vi "Create.vi"(8 "error in (no error)":errorcluster, 10 "Subsystem Name (optional)":string, 11 "SMO":refnum<class "SMO.lvclass">) -> (0 "error out":errorcluster, 2 "SMO name":string, 3 "SMO out":refnum<class "SMO.lvclass">)   [LabVIEW 2013, in "SMO.lvclass"]
doc: "Constructor\n\nNote 01: This method is overridable by descendant\nNote 02: When overridden, Call Parent Method is required\n\n---------------------------------------------------------------\nJKI State Machine Objects™\nhttp://jki.net/state-machine-objects/\nCopyright (C) 2005-2015, JKI <info@jki.net>\nALL RIGHTS RESERVED"
uses:
  SMO.lvclass
  SMO.lvclass/SMO.ctl
  Typedefs/Process Error Notification--Cluster.ctl
  Typedefs/SMOState --Enum.ctl
  Registry/Registry-SMO.lvclass
  Support/Attribute.Identity/Attribute.Identity.lvclass
panel:
  # "For instructions on how to use the JKI State Machine Objects, examples and video tutorials, visit:\nhttp://jki.net/state-machine-objects/\n\nJKI State Machine Objects™\nhttp://jki.net/state-machine-objects/\nCopyright (C) 2005-2015, JKI <info@jki.net>\nALL RIGHTS RESERVED"
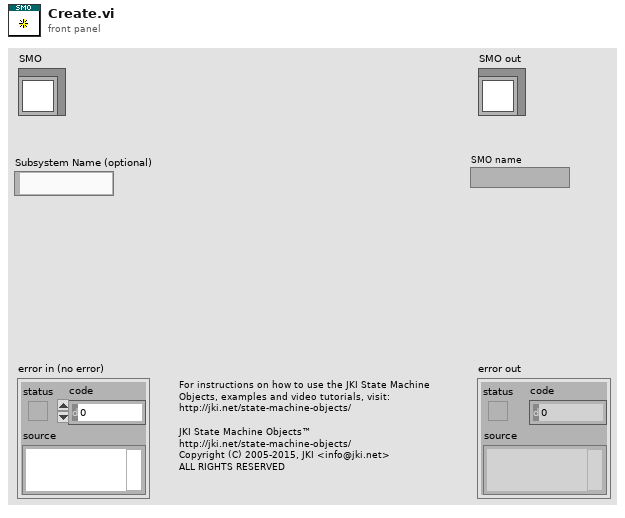
[diagram p1: front panel]
types:
  T1 = typedef "SMO.lvclass/SMOState --Enum.ctl" = enum16{"unknown", "Created", "Started", "Stopped"}
  T2 = typedef "SMO.lvclass/Process Error Notification--Cluster.ctl" = cluster{"error":errorcluster}
  T3 = typedef "SMO.lvclass/PrivateData--Ref.ctl" = refnum<data-value>
  T4 = typedef "SMO.lvclass/PrivateData--Cluster.ctl" = cluster{"Parent Call":T5, "Registered Processes":T6[], "Sync Notifier":refnum<notifier>, "Process Error Notifier":refnum<notifier>, "Protected Events":T7, "Public Events":T8, "SMO State":T1, "[Dependencies]":T9[], "[Attributes]":refnum<class "Attribute.lvclass">[]}
  T5 = typedef "SMO.lvclass/Parent Call--Enum.ctl" = enum16{"Allows parent to run", "Does not request parent to run"}
  T6 = typedef "SMO.lvclass/RegisteredProcessData--Cluster.ctl" = cluster{"Name":string, "Static VI Ref":refnum<vi>, "Running":bool, "NotifierRef":u32}
  T7 = typedef "SMO.lvclass/Protected Events.ctl" = cluster{"StopProcesses":refnum<user-event>, "AbortProcesses":refnum<user-event>}
  T8 = typedef "SMO.lvclass/Public Events.ctl" = cluster{"Error":refnum<user-event>, "State":refnum<user-event>}
  T9 = typedef "SMO.lvclass/SMO Dependency--Cluster.ctl" = cluster{"Dependency":refnum<class "SMO.lvclass">, "Level":string}
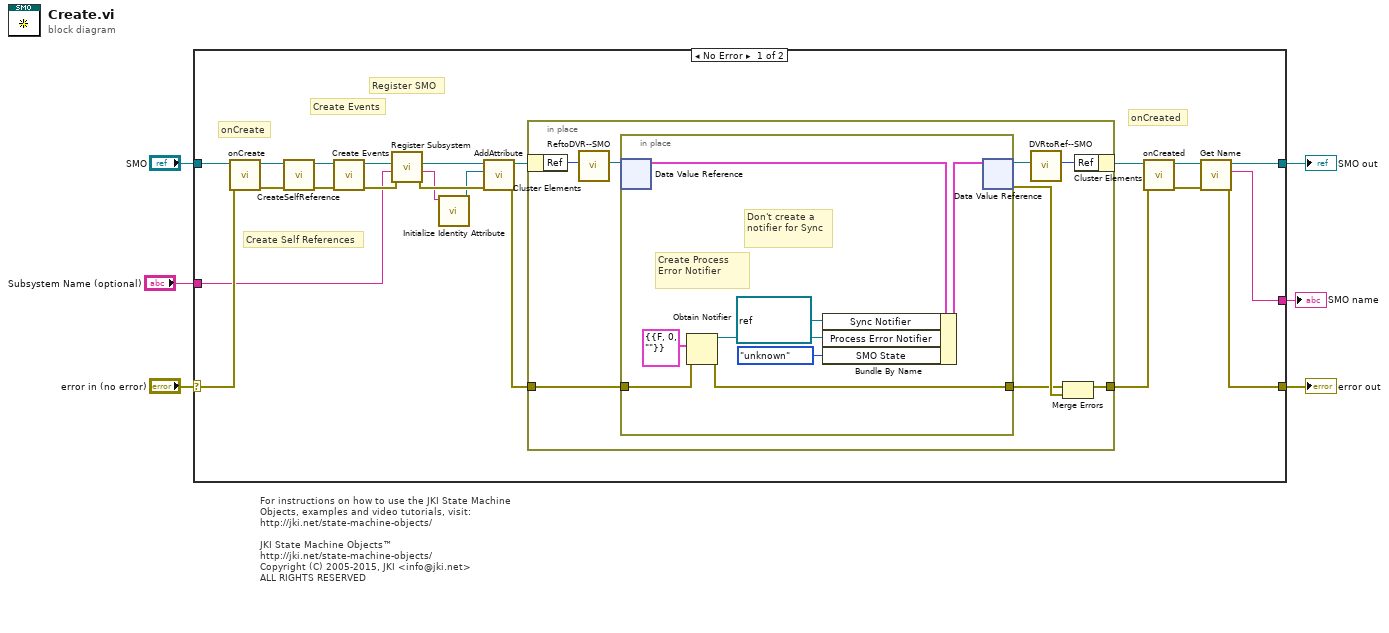
[diagram p0: block diagram]
diagram:
  # "For instructions on how to use the JKI State Machine Objects, examples and video tutorials, visit:\nhttp://jki.net/state-machine-objects/\n\nJKI State Machine Objects™\nhttp://jki.net/state-machine-objects/\nCopyright (C) 2005-2015, JKI <info@jki.net>\nALL RIGHTS RESERVED"
  n1 = case shown="No Error" "error in (no error)" {
    selector: "error in (no error)" -> [w23 w46]
    tunnel: [w18 w46] -> w5
    tunnel: [w20 w45] -> w3
    tunnel: "SMO" -> [w24 w45]
    tunnel: "Subsystem Name (optional)" -> [w22 _]
    tunnel: [w17 _] -> w1
    frame No Error {
      # "Create Self References"
      # "onCreated"
      # "Register SMO"
      # "Create Events"
      # "onCreate"
      n2 = call-dynamic "onCreate.vi"("error in (no error)"=w23, "SMO"=w24) -> ("error out"=w8:errorcluster, "SMO out"=w10:refnum<class "SMO.lvclass">)  [unwired: 8 in]
      n3 = call-dynamic "CreateSelfReference.vi"("error in (no error)"=w8, "SMO"=w10) -> ("error out"=w7:errorcluster, "SMO out"=w9:refnum<class "SMO.lvclass">)  [unwired: 8 in]
      n4 = call "Create Events.vi"("error in (no error)"=w7, "SMO"=w9) -> ("error out"=w27:errorcluster, "SMO out"=w28:refnum<class "SMO.lvclass">)  [unwired: 8 in]
      n5 = call "Register Subsystem.vi"("error in (no error)"=w27, "Subsystem Name (optional)"=w22, "JKI SMO in"=w28) -> ("error out"=w14:errorcluster, "Unique Subsystem Name"=w12:string, "JKI SMO out"=w16:refnum<class "SMO.lvclass">)  [unwired: 6 in]
      n6 = call "Initialize Identity Attribute.vi"("Name"=w12) -> ("Attribute.Identity"=w11:refnum<class "Attribute.Identity.lvclass">)  [unwired: 10 in]
      n7 = call "AddAttribute.vi"("error in (no error)"=w14, "Attribute"=w11, "SMO in"=w16) -> ("error out"=w13:errorcluster, "SMO out"=w15:refnum<class "SMO.lvclass">)  [unwired: 7 in]
      n8 = in-place {
        in-place-border: [w35] -> w25
        in-place-border: w13 -> [w33]
        n9 = in-place-cluster #1(w15) -> ("Ref"=w32:u32)
        n10 = call "ReftoDVR--SMO.vi"("Ref"=w32) -> ("Ref"=w31:T3)  [unwired: 10 in]
        n11 = in-place {
          in-place-border: [w42] -> w34
          in-place-border: w33 -> [w39]
          # "Don't create a notifier for Sync"
          # "Create Process Error Notifier"
          n12 = in-place-dvr #2(w31) -> (w44:T4)  [unwired: 1 out]
          n13 = Obtain Notifier(notification data type=T2 {"error"={"status"=FALSE, "code"=0, "source"=""}} ("Process Notification"), error in (no error)=w39) -> (notifier out=w41:refnum<notifier>, error out=w42:errorcluster)  [unwired: 2 in, 1 out]
          n14 = Bundle By Name(cluster=w44, "Sync Notifier"=refnum<notifier> refnum, "Process Error Notifier"=w41, "SMO State"=SMOState_--Enum."unknown") -> (w43:T4)
          n15 = in-place-dvr #2(w43) -> (w30:T3, w36:errorcluster)
        }
        n16 = call "DVRtoRef--SMO.vi"("Ref"=w30) -> ("Ref"=w29:u32)  [unwired: 10 in]
        n17 = Merge Errors(w34, w36) -> (w35:errorcluster)
        n18 = in-place-cluster #1("Ref"=w29) -> (w26:refnum<class "SMO.lvclass">)
      }
      n19 = call-dynamic "onCreated.vi"("error in (no error)"=w25, "SMO"=w26) -> ("error out"=w19:errorcluster, "SMO out"=w21:refnum<class "SMO.lvclass">)  [unwired: 8 in]
      n20 = call "Get Name.vi"("error in (no error)"=w19, "SMO"=w21) -> ("error out"=w18:errorcluster, "Name"=w17:string, "SMO out"=w20:refnum<class "SMO.lvclass">)  [unwired: 7 in]
    }
    frame Error {
    }
  }
  "error out" <- w5
  "SMO out" <- w3
  "SMO name" <- w1
